vi "Add Waveform.vi"(8 "error in":errorcluster, 10 "Waveforms UI Ctrl Ref":T2, 11 "Waveform Meas Config Ctrl Ref":T1) -> (0 "error out":errorcluster)   [LabVIEW 2025, in "Fgen Script Mode UI.lvlib"]
uses:
  Fgen Script Mode UI.lvlib
  Typedef/Wfm Typedef.ctl
  Typedef/Waveforms UI Ctrl Ref.ctl
  Typedef/Waveform Meas Config Ctrl Ref.ctl
panel:
  in  "Auto Name?":bool=TRUE
  in  "New Wfm Name in Script":string
  in  "Waveform Selection":i32(listbox)
  out "Selected Waveform Preview":waveform(dbl)(graph)
  in  "File Path":path
  in  "Cancel":bool
  in  "OK":bool
  # "* After configure the TDMS file path, select one waveform from the Waveform Selection to add and press OK."
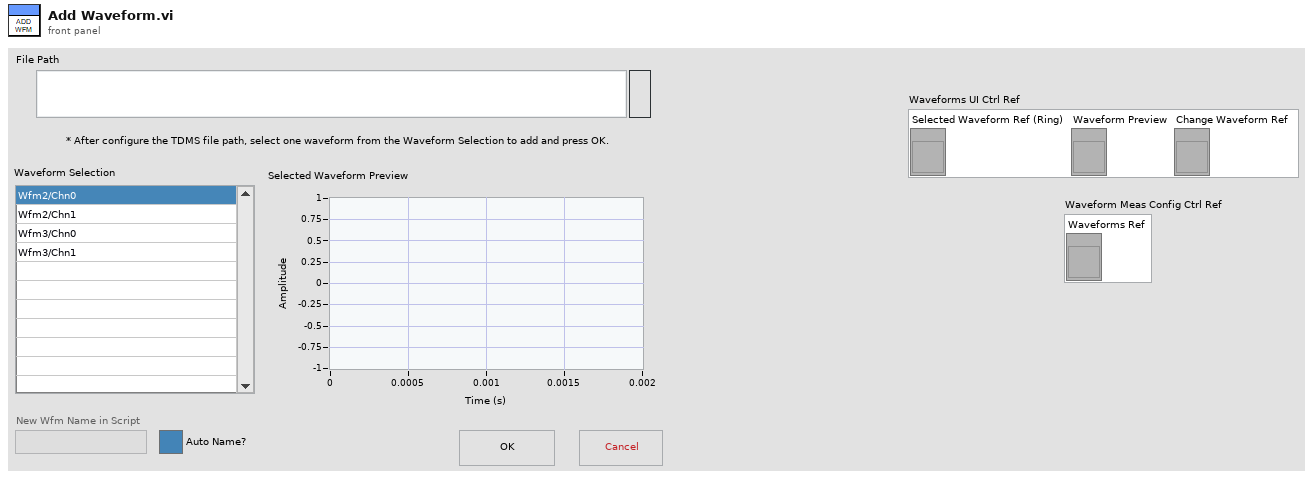
[diagram p1: front panel]
types:
  T1 = typedef "Fgen Script Mode UI.lvlib/Waveform Meas Config Ctrl Ref.ctl" = cluster{"Waveforms Ref":refnum<vi>}
  T2 = typedef "Fgen Script Mode UI.lvlib/Waveforms UI Ctrl Ref.ctl" = cluster{"Selected Waveform Ref (Ring)":refnum<vi>, "Waveform Preview":refnum<vi>, "Change Waveform Ref":refnum<vi>}
  T3 = typedef "Fgen Script Mode UI.lvlib/Wfm Typedef.ctl" = cluster{"Name":string, "Path":string, "Grp":string, "Chn":string}
  T4 = enum8{"Enabled", "Disabled", "Disabled and Grayed Out"}
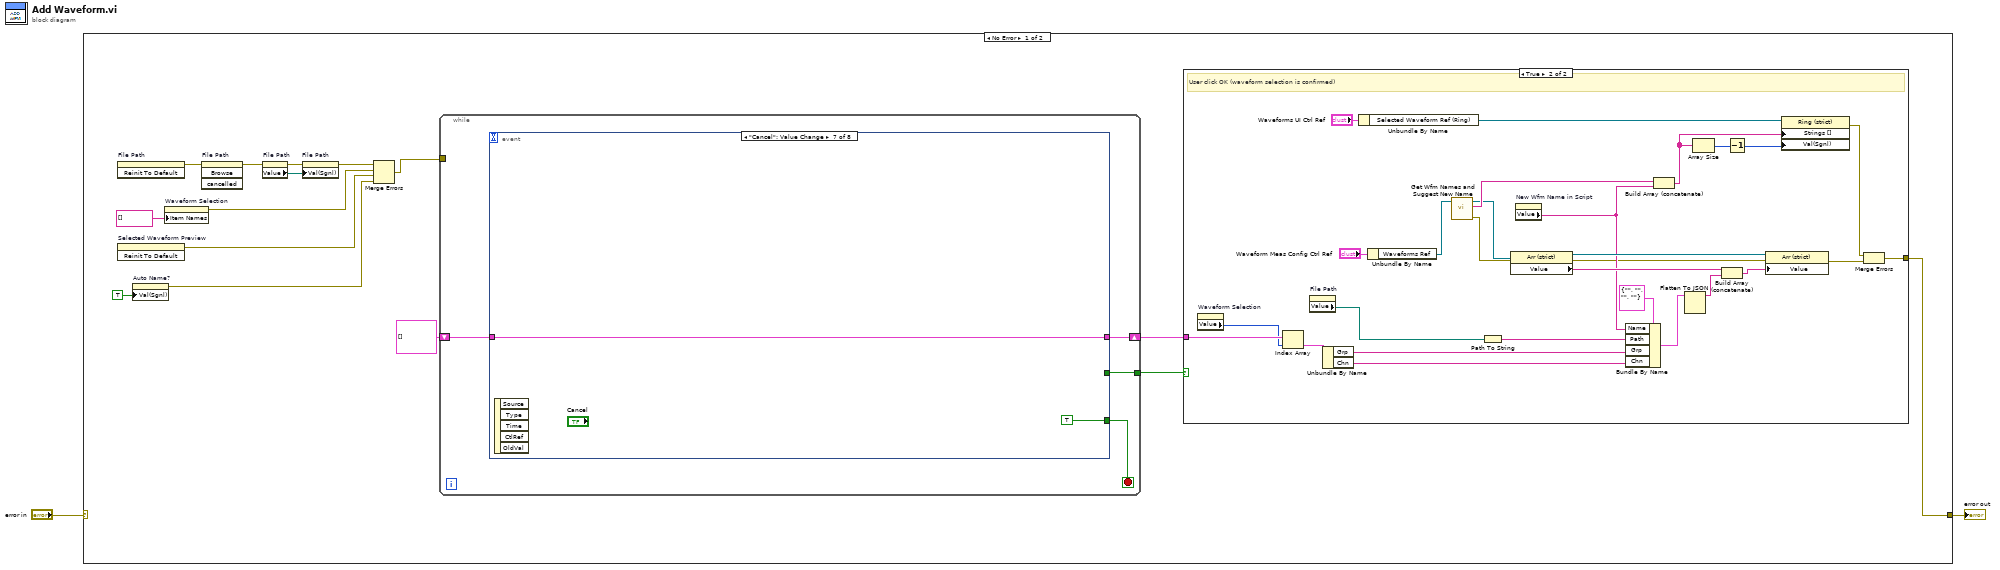
[diagram p0: block diagram]
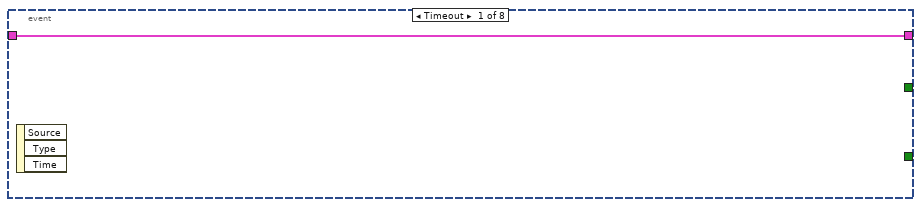
[diagram p3: hidden frame]
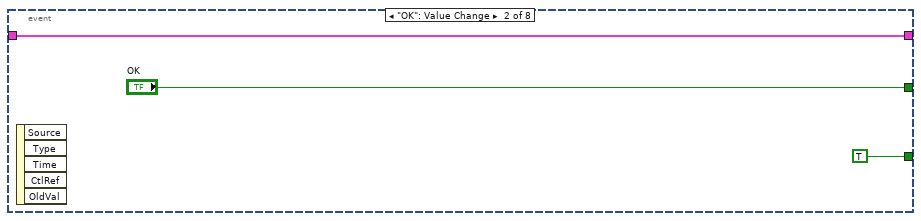
[diagram p4: hidden frame]
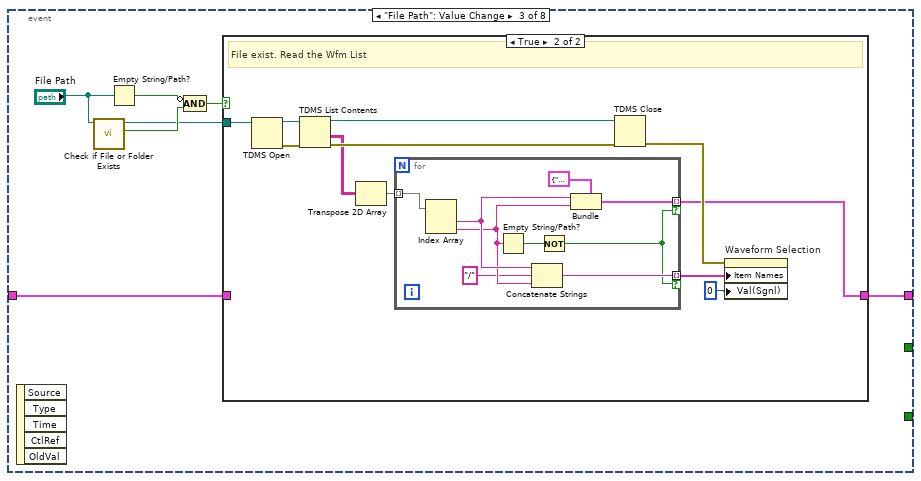
[diagram p5: hidden frame]
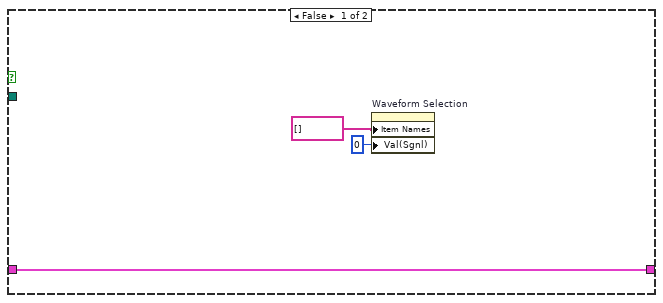
[diagram p6: hidden frame]
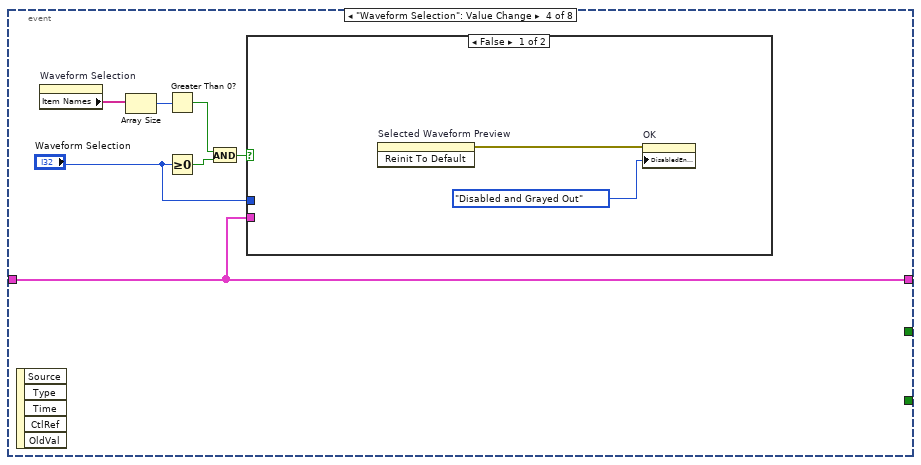
[diagram p7: hidden frame]
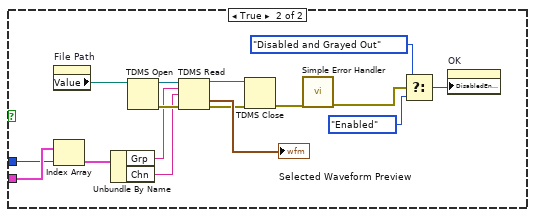
[diagram p8: hidden frame]
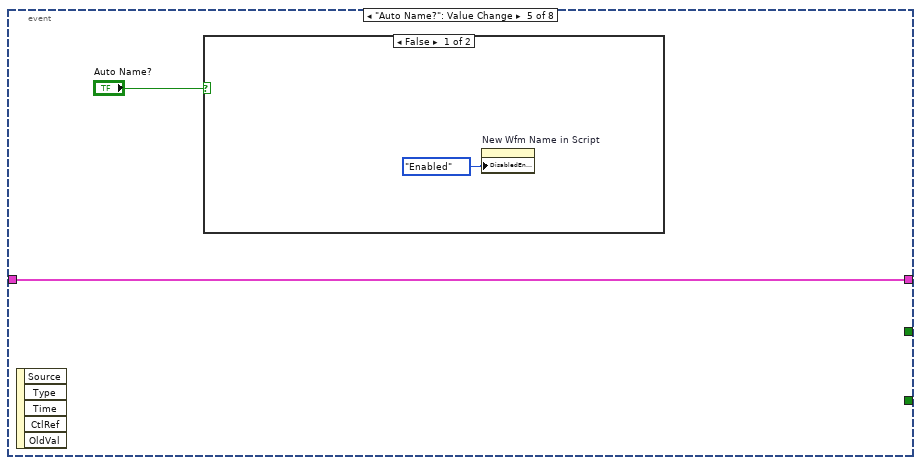
[diagram p9: hidden frame]
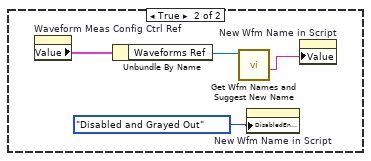
[diagram p10: hidden frame]
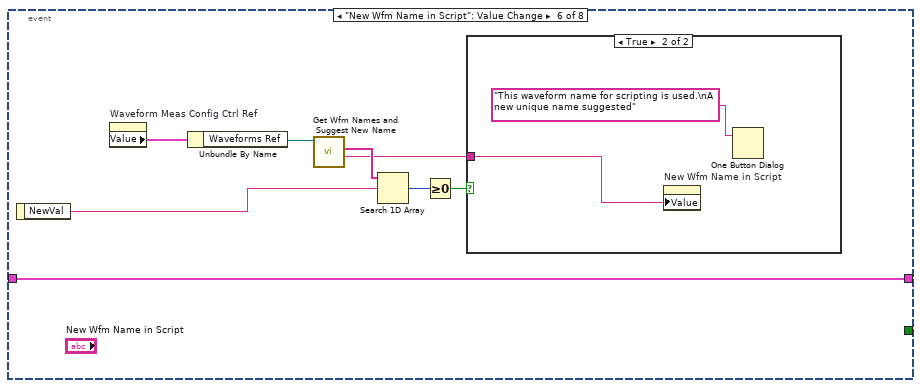
[diagram p11: hidden frame]
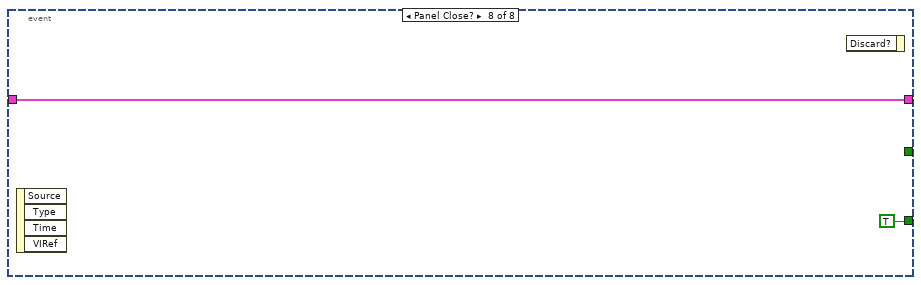
[diagram p13: hidden frame]
diagram:
  n1 = case shown="No Error" "error in" {
    selector: "error in" -> [_ w130]
    tunnel: [w5 w130] -> w1
    frame No Error {
      n2 = invoke on="File Path" class="Path" method="Reinit To Default"() -> (error out=w17:errorcluster)  [unwired: 3 in, 2 out]
      n3 = invoke on="Selected Waveform Preview" class="WFGraph (strict)" method="Reinit To Default"() -> (error out=w8:errorcluster)  [unwired: 3 in, 2 out]
      n4 = property on="Auto Name?" class="Bool (strict)"("Val(Sgnl)"=TRUE ("Value (Signaling)")) -> (error out=w4:errorcluster)  [unwired: 2 in, 1 out]
      n5 = property on="Waveform Selection" class="LstBox (strict)"("Item Names"=string[] []) -> (error out=w9:errorcluster)  [unwired: 2 in, 1 out]
      n6 = invoke on="File Path" class="Path" method="Browse"(error in=w17) -> (error out=w15:errorcluster)  [unwired: 3 in, 3 out]
      n7 = property on="File Path" class="Path"(error in=w15) -> (error out=w13:errorcluster, "Value"=w14:path)  [unwired: 1 in, 1 out]
      n8 = property on="File Path" class="Path"(error in=w13, "Val(Sgnl)"=w14) -> (error out=w12:errorcluster)  [unwired: 1 in, 1 out]
      n9 = Merge Errors(w12, w9, w8, w4) -> (w10:errorcluster)
      n10 = while {
        tunnel: w10 -> [_]
        shift-right: [w48] -> w6
        shift-left: cluster{"Grp":string, "Chn":string}[] [] -> [w47]
        tunnel: [w46] -> w7
        stop <- w49 stop-if-true
        n11 = event shown="[6] \"Cancel\": Value Change" {
          selector: _ -> [_ _ _ _ _ _ _ _]
          dyn-events: _ -> [_ _ _ _ _ _ _ _]
          timeout: _ -> [_ _ _ _ _ _ _ _]
          tunnel: [_ "OK" _ _ _ _ _ _] -> w46
          tunnel: [_ TRUE _ _ _ _ TRUE TRUE] -> w49
          tunnel: [w50 w51 w55 w85 w110 w123 w126 w129] -> w48
          tunnel: w47 -> [w50 w51 w54 w85 w110 w123 w126 w129]
          event Timeout {
            n12 = event-data() -> ()  [unwired: 1 in, 3 out]
          }
          event "OK": Value Change {
            n13 = event-data() -> ()  [unwired: 1 in, 5 out]
          }
          event "File Path": Value Change {
            n14 = event-data() -> ()  [unwired: 1 in, 5 out]
            n15 = call <vilib>:"Check if File or Folder Exists.vi"("path"="File Path") -> ("file or folder exists?"=w58:bool, "dup path"=w56:path)  [unwired: 8 in, 1 out]
            n16 = Empty String/Path?(string/path="File Path") -> (empty?=w59:bool)
            n17 = Compound Arithmetic op=AND(invert w59, w58) -> (w57:bool)
            n18 = case shown="True" w57 {
              tunnel: w56 -> [_ w74]
              tunnel: [w63 w65] -> w55
              tunnel: w54 -> [w63 _]
              frame False {
                n19 = property on="Waveform Selection" class="LstBox (strict)"("Item Names"=string[] [], "Val(Sgnl)"=0 ("Waveform Selection")) -> ()  [unwired: 2 in, 2 out]
              }
              frame True {
                # "File exist. Read the Wfm List"
                n20 = TDMS Open(11:w74) -> (0:w73:errorcluster, 3:w72:refnum<k34>)  [unwired: 6 in]
                n21 = TDMS List Contents(4:w73, 7:w72) -> (0:w70:errorcluster, 1:w68:string[][], 3:w71:refnum<k34>)  [unwired: 1 in, 1 out]
                n22 = Transpose 2D Array(2D array=w68) -> (transposed array=w69:string[][])
                n23 = for {
                  tunnel: w69 -> [w83] mode=indexing
                  tunnel: [w80] -> w65 mode=indexing if=w75
                  tunnel: [w76] -> w67 mode=indexing if=w75
                  n24 = Index Array(array=w83) -> (element #1=w79:string, element #2=w78:string)  [unwired: 2 in]
                  n25 = Empty String/Path?(string/path=w78) -> (empty?=w82:bool)
                  n26 = Concatenate Strings(w79, "/" ("string"), w78) -> (w76:string)
                  n27 = Not(x=w82) -> (.not. x?=w75:bool)
                  n28 = Bundle(cluster=cluster{"Grp":string, "Chn":string} {"Grp"="", "Chn"=""} ("output cluster"), "Grp"=w79, "Chn"=w78) -> (w80:cluster{"Grp":string, "Chn":string})
                }
                n29 = TDMS Close(8:w70, 11:w71) -> (0:w66:errorcluster)  [unwired: 1 out]
                n30 = property on="Waveform Selection" class="LstBox (strict)"(error in=w66, "Item Names"=w67, "Val(Sgnl)"=0 ("Waveform Selection")) -> ()  [unwired: 1 in, 2 out]
              }
            }
          }
          event "Waveform Selection": Value Change {
            n31 = event-data() -> ()  [unwired: 1 in, 5 out]
            n32 = property on="Waveform Selection" class="LstBox (strict)"() -> ("Item Names"=w89:string[])  [unwired: 2 in, 2 out]
            n33 = Array Size(array=w89) -> (size(s)=w88:i32)
            n34 = Greater Than 0?(x=w88) -> (x > 0?=w86:bool)
            n35 = Greater Or Equal To 0?(x="Waveform Selection") -> (x >= 0?=w90:bool)
            n36 = And(x=w86, y=w90) -> (x .and. y?=w87:bool)
            n37 = case shown="False" w87 {
              tunnel: w85 -> [_ w107]
              tunnel: "Waveform Selection" -> [_ w106]
              frame False {
                n38 = invoke on="Selected Waveform Preview" class="WFGraph (strict)" method="Reinit To Default"() -> (error out=w92:errorcluster)  [unwired: 3 in, 2 out]
                n39 = property on="OK" class="Bool"(error in=w92, "DisabledEnum"=T4."Disabled and Grayed Out" ("Disabled")) -> ()  [unwired: 1 in, 2 out]
              }
              frame True {
                n40 = property on="File Path" class="Path"() -> ("Value"=w108:path)  [unwired: 2 in, 2 out]
                n41 = Index Array(array=w107, index=w106) -> (element=w103:cluster{"Grp":string, "Chn":string})
                n42 = Unbundle By Name(w103) -> ("Grp"=w102:string, "Chn"=w101:string)
                n43 = TDMS Open(11:w108) -> (0:w104:errorcluster, 3:w105:refnum<k34>)  [unwired: 6 in]
                n44 = TDMS Read(0:w105, 5:w102, 7:w101, 11:w104) -> (4:w99:refnum<k34>, 10:→"Selected Waveform Preview":waveform(dbl), 15:w98:errorcluster)  [unwired: 4 in, 3 out]
                n45 = TDMS Close(8:w98, 11:w99) -> (0:w97:errorcluster)  [unwired: 1 out]
                n46 = call <vilib>:"Simple Error Handler.vi"("error in (no error)"=w97) -> ("error out"=w96:errorcluster)  [unwired: 4 in, 4 out]
                n47 = Select(t=T4."Disabled and Grayed Out" ("Disabled"), s=w96, f=T4."Enabled" ("Disabled")) -> (s? t:f=w93:T4)
                n48 = property on="OK" class="Bool"("DisabledEnum"=w93) -> ()  [unwired: 2 in, 2 out]
              }
            }
          }
          event "Auto Name?": Value Change {
            n49 = event-data() -> ()  [unwired: 1 in, 5 out]
            n50 = case shown="False" "Auto Name?" {
              frame False {
                n51 = property on="New Wfm Name in Script" class="Str"("DisabledEnum"=T4."Enabled" ("Disabled")) -> ()  [unwired: 2 in, 2 out]
              }
              frame True {
                n52 = property on="Waveform Meas Config Ctrl Ref" class="Clust (strict)"() -> ("Value"=w115:T1)  [unwired: 2 in, 2 out]
                n53 = Unbundle By Name(w115) -> ("Waveforms Ref"=w114:refnum<vi>)
                n54 = call "Get Wfm Names and Suggest New Name.vi"("Wfm Ref In"=w114) -> ("New Wfm Name"=w113:string)  [unwired: 7 in, 3 out]
                n55 = property on="New Wfm Name in Script" class="Str"("DisabledEnum"=T4."Disabled and Grayed Out" ("Disabled")) -> ()  [unwired: 2 in, 2 out]
                n56 = property on="New Wfm Name in Script" class="Str"("Value"=w113) -> ()  [unwired: 2 in, 2 out]
              }
            }
          }
          event "New Wfm Name in Script": Value Change {
            n57 = event-data() -> ("NewVal"=w119:string)  [unwired: 1 in]
            n58 = property on="Waveform Meas Config Ctrl Ref" class="Clust (strict)"() -> ("Value"=w122:T1)  [unwired: 2 in, 2 out]
            n59 = Unbundle By Name(w122) -> ("Waveforms Ref"=w121:refnum<vi>)
            n60 = call "Get Wfm Names and Suggest New Name.vi"("Wfm Ref In"=w121) -> ("New Wfm Name"=w116:string, "Wfm Names"=w120:string[])  [unwired: 7 in, 2 out]
            n61 = Search 1D Array(1D array=w120, element=w119) -> (index of element=w118:i32)  [unwired: 1 in]
            n62 = Greater Or Equal To 0?(x=w118) -> (x >= 0?=w117:bool)
            n63 = case shown="True" w117 {
              tunnel: w116 -> [_ w124]
              frame False {
              }
              frame True {
                n64 = property on="New Wfm Name in Script" class="Str"("Value"=w124) -> ()  [unwired: 2 in, 2 out]
                n65 = One Button Dialog(message="This waveform name for scripting is used.\nA new unique name suggested") -> ()  [unwired: 1 in, 1 out]
              }
            }
          }
          event "Cancel": Value Change {
            n66 = event-data() -> ()  [unwired: 1 in, 5 out]
          }
          event Panel Close? {
            n67 = event-data() -> ()  [unwired: 1 in, 4 out]
            n68 = event-data() -> ()  [unwired: 2 in, 1 out]
          }
        }
      }
      n69 = case shown="True" w7 {
        tunnel: w6 -> [_ w45]
        tunnel: [_ w28] -> w5
        frame False {
        }
        frame True {
          # "User click OK (waveform selection is confirmed)"
          n70 = property on="Waveform Selection" class="LstBox (strict)"() -> ("Value"=w44:i32)  [unwired: 2 in, 2 out]
          n71 = Index Array(array=w45, index=w44) -> (element=w40:cluster{"Grp":string, "Chn":string})
          n72 = property on="File Path" class="Path"() -> ("Value"=w41:path)  [unwired: 2 in, 2 out]
          n73 = Unbundle By Name(w40) -> ("Grp"=w39:string, "Chn"=w38:string)
          n74 = Unbundle By Name("Waveforms UI Ctrl Ref") -> ("Selected Waveform Ref (Ring)"=w32:refnum<vi>)
          n75 = Unbundle By Name("Waveform Meas Config Ctrl Ref") -> ("Waveforms Ref"=w37:refnum<vi>)
          n76 = call "Get Wfm Names and Suggest New Name.vi"("Wfm Ref In"=w37) -> ("error out"=w19:errorcluster, "Wfm Names"=w25:string[], "Wfm Ref Out"=w23:refnum<vi>)  [unwired: 7 in, 1 out]
          n77 = Path To String(path=w41) -> (string=w42:string)
          n78 = property class="Arr (strict)"(reference=w23, error in=w19) -> (reference out=w22:refnum<vi>, error out=w18:errorcluster, "Value"=w21:string[])
          n79 = property on="New Wfm Name in Script" class="Str"() -> ("Value"=w20:string)  [unwired: 2 in, 2 out]
          n80 = Bundle By Name(cluster=T3 {"Name"="", "Path"="", "Grp"="", "Chn"=""} ("Waveform"), "Name"=w20, "Path"=w42, "Grp"=w39, "Chn"=w38) -> (w36:T3)
          n81 = Build Array (concatenate)(w25, w20) -> (w24:string[])
          n82 = Flatten To JSON(anything=w36) -> (JSON string=w35:string)  [unwired: 2 in, 1 out]
          n83 = Array Size(array=w24) -> (size(s)=w31:i32)
          n84 = Build Array (concatenate)(w21, w35) -> (w27:string[])
          n85 = Decrement(x=w31) -> (x-1=w26:i32)
          n86 = property class="Arr (strict)"(reference=w22, error in=w18, "Value"=w27) -> (error out=w30:errorcluster)  [unwired: 1 out]
          n87 = property class="Ring (strict)"(reference=w32, "Strings []"=w24, "Val(Sgnl)"=w26) -> (error out=w29:errorcluster)  [unwired: 1 in, 1 out]
          n88 = Merge Errors(w29, w30) -> (w28:errorcluster)
        }
      }
    }
    frame Error {
    }
  }
  "error out" <- w1
